vi "Convert Milliseconds to Time.vi"(0 "milliseconds":u32) -> (1 "elapsed time":string)   [LabVIEW 2010]
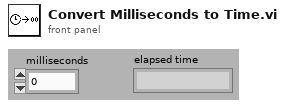
[diagram p1: front panel]
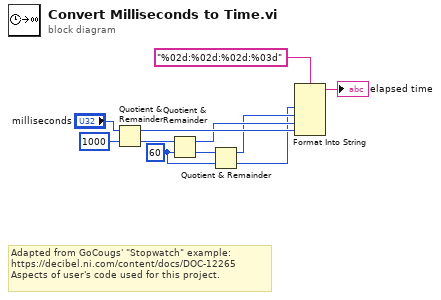
[diagram p0: block diagram]
diagram:
  w9 = u32 60 ("y")
  # "Adapted from GoCougs' \"Stopwatch\" example:\nhttps://decibel.ni.com/content/docs/DOC-12265\nAspects of user's code used for this project."
  n1 = Quotient & Remainder(x="milliseconds", y=u32 1000) -> (x-y*floor(x/y)=w7:u32, floor(x/y)=w10:u32)
  n2 = Quotient & Remainder(x=w10, y=w9) -> (x-y*floor(x/y)=w6:u32, floor(x/y)=w8:u32)
  n3 = Quotient & Remainder(x=w8, y=w9) -> (x-y*floor(x/y)=w5:u32, floor(x/y)=w4:u32)
  n4 = Format Into String(format string="%02d:%02d:%02d:%03d", w4, w5, w6, w7) -> (resulting string=→"elapsed time":string)  [unwired: 2 in, 1 out]
